vi "Control Engine.vi"(7 "All References":refnum<vi>[](array[refnum]), 8 "error in (no error)":errorcluster, 9 "Matched controls":refnum<vi>[](array[refnum]), 10 "Rules":T1[](array[typedef]), 11 "Event Registration Refnum in":refnum<event-registration>) -> (0 "error out":errorcluster)   [LabVIEW 2019, in "LSS.lvlib"]
doc: "This is the property control engine. It launches asynchronously and runs in the background. Using the events registered for by the launcher it monitores controls based on the rules input and will stylize them using the effects input when the criteria are met. \n\n<b>Inputs:</b>\n<b>All References</b> - List of all objects that can be stylized using LSS from the front panel of the VI to be controlled.\n<b>Event Registration Refnum in</b> - Contains the registered value change events for the controls that will be effected by the criteria.\n<b>Rules</b> - List of rules that will be monitored, when their conditions are met, their effecs will be applied.\n<b>Relevent Controls</b> - List of controls whose refnums are registered. This list is used as a reference point into the list of Rules when events are fired.\n<b>Error In</b> - Standard Error In terminal.\n\n<b>Outputs:</b>\n<b>Error Out</b> - Standard Error out terminal."
uses:
  LSS.lvlib
  Controls/Rule.ctl
  Controls/Criteria.ctl
  Controls/Comparison Types.ctl
  Controls/Effects.ctl
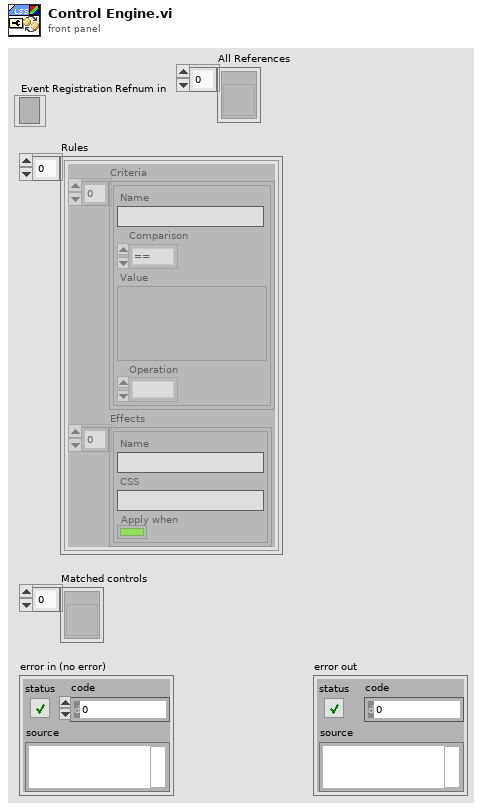
[diagram p1: front panel]
types:
  T1 = typedef "LSS.lvlib/Rule.ctl" = cluster{"Criteria":T2[], "Effects":T4[]}
  T2 = typedef "LSS.lvlib/Criteria.ctl" = cluster{"Name":string, "Comparison":T3, "Value":variant, "Operation":enum16{"Stack", "&&", "||"}}
  T3 = typedef "LSS.lvlib/Comparison Types.ctl" = enum16{"==", "!=", "<", ">", "<=", ">="}
  T4 = typedef "LSS.lvlib/Effects.ctl" = cluster{"Name":string, "CSS":string, "Apply when":bool}
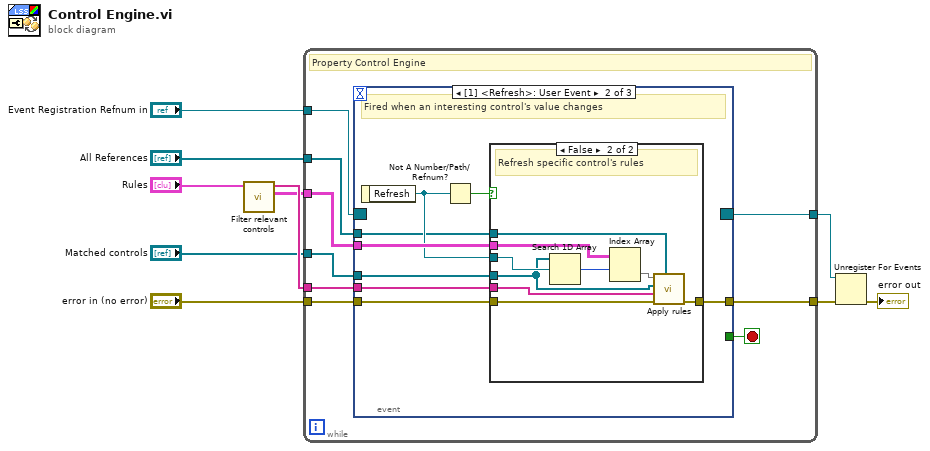
[diagram p0: block diagram]
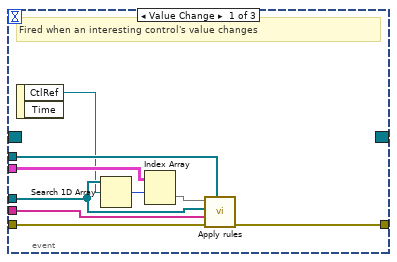
[diagram p2: hidden frame]
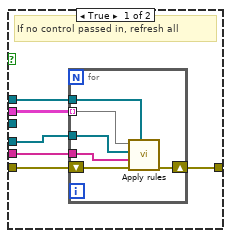
[diagram p3: hidden frame]
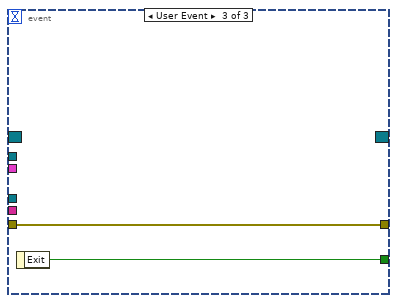
[diagram p4: hidden frame]
diagram:
  n1 = call "Filter relevant controls.vi"("Rules"="Rules") -> ("Relevant Rules"=w8:T1[][], "Relevent Controls"=w10:string[])  [unwired: 9 in]
  n2 = while {
    tunnel: "Event Registration Refnum in" -> [w19]
    tunnel: "Matched controls" -> [w18]
    tunnel: w8 -> [w17]
    tunnel: w10 -> [w16]
    tunnel: [w14] -> w5
    tunnel: "All References" -> [w13]
    tunnel: "error in (no error)" -> [w15]
    tunnel: [w11] -> w7
    stop <- w12 stop-if-true
    # "Property Control Engine"
    n3 = event shown="[1] <Refresh>: User Event" {
      selector: w19 -> [_ _ _]
      dyn-events: [_ _ _] -> w14
      timeout: _ -> [_ _ _]
      tunnel: [_ _ w58] -> w12
      tunnel: w18 -> [w26 w34 _]
      tunnel: w17 -> [w28 w36 _]
      tunnel: w16 -> [w27 w35 _]
      tunnel: w15 -> [w25 w33 w59]
      tunnel: [w24 w32 w59] -> w11
      tunnel: w13 -> [w23 w29 _]
      event Value Change {
        # "Fired when an interesting control's value changes"
        n4 = event-data() -> ("CtlRef"=w22:refnum<vi>)  [unwired: 1 in, 1 out]
        n5 = Search 1D Array(1D array=w26, element=w22) -> (index of element=w20:i32)  [unwired: 1 in]
        n6 = Index Array(array=w28, index (row)=w20) -> (element=w21:T1[])  [unwired: 1 in]
        n7 = call "Apply rules.vi"("All References"=w23, "Error in"=w25, "Relevant control names"=w27, "Relevant controls"=w26, "Rules to apply"=w21) -> ("Error out"=w24:errorcluster)  [unwired: 4 in]
      }
      event User Event {
        # "Fired when an interesting control's value changes"
        n8 = event-data() -> ("Refresh"=w31:refnum<vi>)  [unwired: 1 in]
        n9 = Not A Number/Path/Refnum?(number/path/refnum=w31) -> (NaN/Path/Refnum?=w30:bool)
        n10 = case shown="False" w30 {
          tunnel: w31 -> [_ w57]
          tunnel: w36 -> [w38 w56]
          tunnel: w35 -> [w42 w54]
          tunnel: w34 -> [w41 w53]
          tunnel: w33 -> [w40 w51]
          tunnel: [w39 w50] -> w32
          tunnel: w29 -> [w37 w49]
          frame True {
            # "If no control passed in, refresh all"
            n11 = for {
              tunnel: w42 -> [w48]
              tunnel: w41 -> [w47]
              shift-right: [w45] -> w39
              shift-left: w40 -> [w46]
              tunnel: w38 -> [w44] mode=indexing
              tunnel: w37 -> [w43]
              n12 = call "Apply rules.vi"("All References"=w43, "Error in"=w46, "Relevant control names"=w48, "Relevant controls"=w47, "Rules to apply"=w44) -> ("Error out"=w45:errorcluster)  [unwired: 4 in]
            }
          }
          frame False {
            # "Refresh specific control's rules"
            n13 = Search 1D Array(1D array=w53, element=w57) -> (index of element=w52:i32)  [unwired: 1 in]
            n14 = Index Array(array=w56, index (row)=w52) -> (element=w55:T1[])  [unwired: 1 in]
            n15 = call "Apply rules.vi"("All References"=w49, "Error in"=w51, "Relevant control names"=w54, "Relevant controls"=w53, "Rules to apply"=w55) -> ("Error out"=w50:errorcluster)  [unwired: 4 in]
          }
        }
      }
      event User Event {
        n16 = event-data() -> ("Exit"=w58:bool)  [unwired: 1 in]
      }
    }
  }
  n17 = Unregister For Events(event registration refnum=w5, error in=w7) -> (error out=→"error out":errorcluster)
